vi "SGUI Assign Single String With Tags.vi"(6 "error in":errorcluster, 8 "string ref":refnum<vi>, 9 "string (empty)":string, 10 "keep last font face setup (False)":bool) -> (7 "error out":errorcluster, 11 "string ref out (copy)":refnum<vi>)   [LabVIEW 2013, in "varilib.lvlib"]
doc: "This VI parses string for tags, assigns the text to the references string object and then sets formats of the text according the tags. It supports multiline strings, i.e. various formats may be selected for each line or even part of the line. Nested tags are supported. If end tag is not found the start tag applies up to end of the whole string.\n\nSupported paired tags:\n <b></b> - bold\n <i></i> - coursive\n <u></u> - underline\n <s></s> - strikeout\n <tc=color></tc> - text color, 'color' is {black;white;red;green;gold;gray;cyan;blue} or hexa number: RRGGBB\n <sz=size></sz> - text size, 'size' is integer\n\nUnpaired tags (global for whole string):\n <bc=color> - background color, no end tag, changes color for entire string object\n <al=mode> - align mode, 'mode' is {left,center,right}\n <keep> - keep last font face setup (b,u,i,s)\n\n<keep> tag or 'keep last font face setup' input will inhibit reset of the font face setup, i.e. if the last used font face was for instance bold, next writting to the stringobject will be in the bold even without any tag specifier.\n\nText color specifier and size are always remembered from last use because default state is unknown. So when multiple sizes or colors were used previously in the string object it is necessary to write start tag with default color/size to start of the line to ensure defined states!\n\nIt ignores input error (executes anyway) however it will generate error if reference writting fails (invalid reference)."
uses:
  varilib.lvlib
  SGUI Assign String With Tags Tag.ctl
  SGUI Assign String With Tags Tag Type.ctl
  <vilib>/Utility/miscctls.llb/LVSelectionTypeDef.ctl
  <vilib>/Utility/error.llb/Error Cluster From Error Code.vi
  <vilib>/regexp/Match Regular Expression.xnode
  <vilib>/ErrorRing/Error Ring.xnode
panel:
  out "Array":bool[][](array[boolean])
  out "tag list":T1[](array[typedef])
  # "Text Tag\n\n<B> Bold </B>\n<I> Italic </I>\n<U> Underline </U>\n<S> Strikeout </S> \n<tc=color></tc> - text color, 'color' is {black;white;red;green;gold;gray;cyan;blue} or hexa number: RRGGBB\n <sz=size></sz> - text size, 'size' is integer\n\nUnpaired tags (global for whole string):\n <bc=color> - background color, no end tag, changes color for entire string object\n <al=mode> - align mode, 'mode' is {left,center,right}\n <keep> - keep last font face setup (b,u,i,s)"
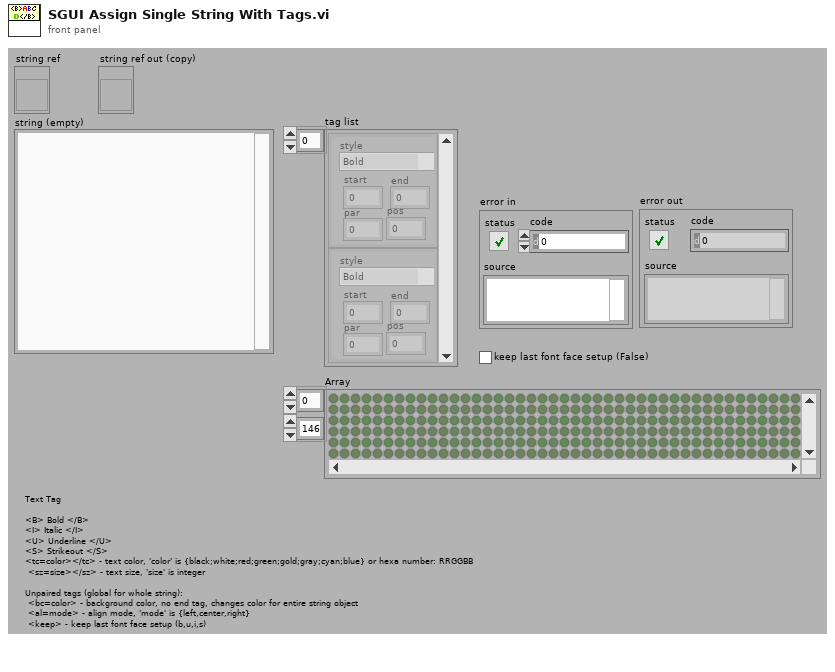
[diagram p1: front panel]
types:
  T1 = typedef "varilib.lvlib/SGUI Assign String With Tags Tag.ctl" = cluster{"pos":i32, "style":T2, "start":i32, "end":i32, "par":i32}
  T2 = typedef "varilib.lvlib/SGUI Assign String With Tags Tag Type.ctl" = enum16{"Bold", "Italic", "Underline", "Strikeout", "Text color", "Bg color", "Align", "Size", "Keep", "n/a"}
  T3 = typedef "LVSelectionTypeDef.ctl" = cluster{"Selection Start":u32, "Selection End":u32}
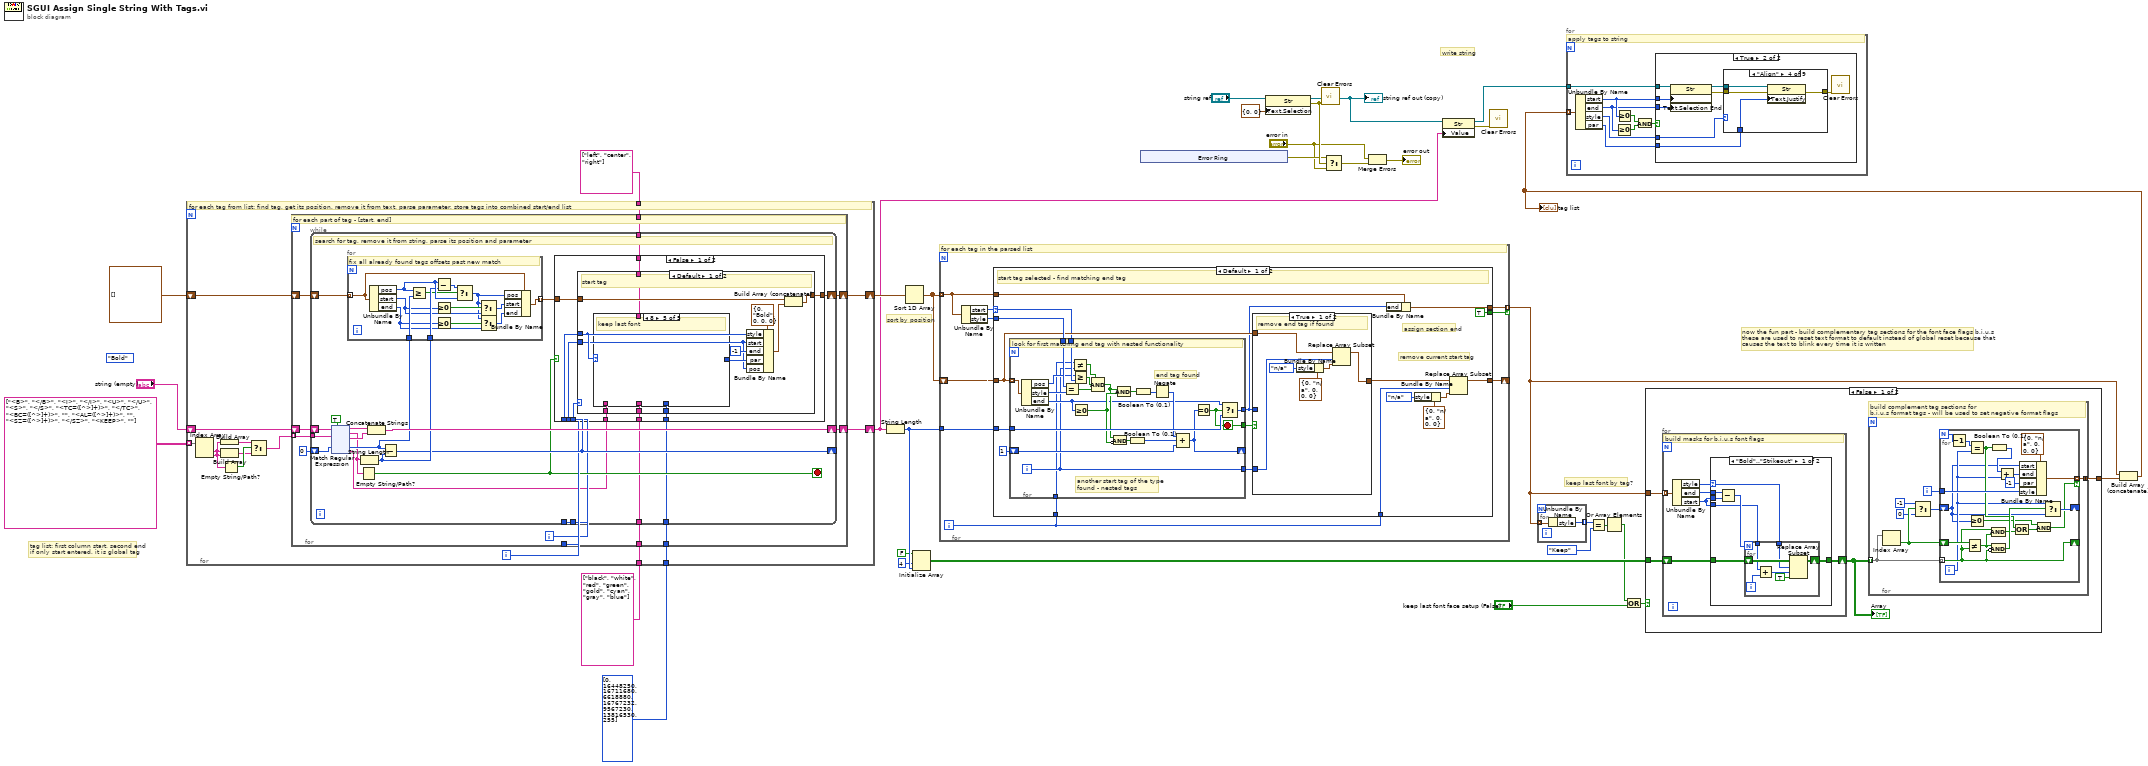
[diagram p0: block diagram]
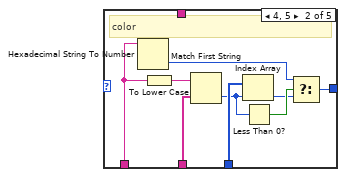
[diagram p7: hidden frame]
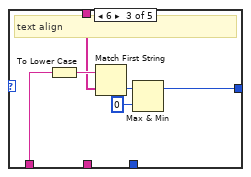
[diagram p8: hidden frame]
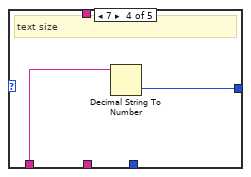
[diagram p9: hidden frame]
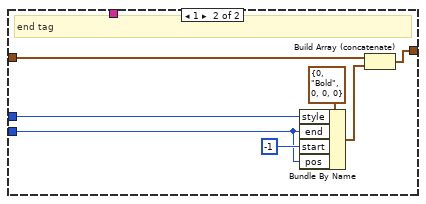
[diagram p10: hidden frame]
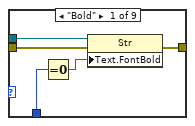
[diagram p13: hidden frame]
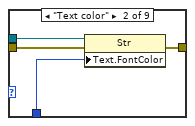
[diagram p14: hidden frame]
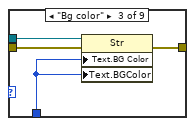
[diagram p15: hidden frame]
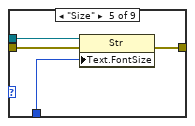
[diagram p16: hidden frame]
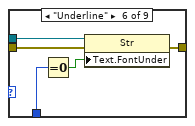
[diagram p17: hidden frame]
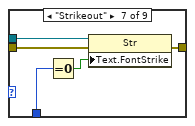
[diagram p18: hidden frame]
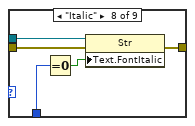
[diagram p19: hidden frame]
diagram:
  (unwired) SGUI_Assign_String_With_Tags_Tag_Type."Bold" ("style")
  # "keep last font by tag?"
  # "now the fun part - build complementary tag sections for the font face flags b,i,u,s\nthese are used to reset text format to default instead of global reset because that\ncauses the text to blink every time it is written"
  # "tag list: first column start, second end\nif only start entered, it is global tag"
  # "write string"
  # "sort by position"
  n1 = for {
    tunnel: string[][] [["<B>", "</B>"], ["<I>", "</I>"], ["<U>", "</U>"], ["<S>", "</S>"], ["<TC=([^>]+)>", "</TC>"], ["<BC=([^>]+)>", ""], ["<AL=([^>]+)>", ""], ["<SZ=([^>]+)>", "</SZ>"], ["<KEEP>", ""]] -> [w46] mode=indexing
    shift-right: [w45] -> w20
    shift-left: "string (empty)" -> [w47]
    shift-right: [w43] -> w25
    shift-left: T1[] [] -> [w44]
    tunnel: string[] ["black", "white", "red", "green", "gold", "cyan", "gray", "blue"] ("string array") -> [w41]
    tunnel: u32[] [0, 16448250, 16711680, 6618880, 16767232, 9567230, 13816530, 255] -> [w40]
    tunnel: string[] ["left", "center", "right"] ("string array") -> [w33]
    i -> [w42]
    # "for each tag from list: find tag, get its position, remove it from text, parse parameter, store tags into combined start/end list"
    n2 = Index Array(array=w46) -> (element #1=w35:string, element #2=w37:string)  [unwired: 2 in]
    n3 = Build Array(w35) -> (w34:string[])
    n4 = Build Array(w35, w37) -> (w36:string[])
    n5 = Empty String/Path?(string/path=w37) -> (empty?=w38:bool)
    n6 = Select(t=w34, s=w38, f=w36) -> (s? t:f=w39:string[])
    n7 = for {
      tunnel: w39 -> [w57] mode=indexing
      tunnel: w42 -> [w53]
      shift-right: [w52] -> w43
      shift-left: w44 -> [w54]
      shift-right: [w56] -> w45
      shift-left: w47 -> [w58]
      tunnel: w41 -> [w50]
      tunnel: w40 -> [w49]
      tunnel: w33 -> [w48]
      i -> [w51]
      # "for each part of tag - [start, end]"
      n8 = while {
        tunnel: w57 -> [w64]
        shift-right: [w70] -> _
        shift-left: 0 -> [w76]
        shift-right: [w77] -> w56
        shift-left: w58 -> [w75]
        shift-right: [w67] -> w52
        shift-left: w54 -> [w73]
        tunnel: w53 -> [w69]
        tunnel: w51 -> [w65]
        tunnel: w50 -> [w61]
        tunnel: w49 -> [w60]
        tunnel: w48 -> [w59]
        stop <- w66 stop-if-true
        # "search for tag, remove it from string, parse its position and parameter"
        n9 = xnode "Match Regular Expression"("input string"=w75, "regular expression"=w64, "offset (0)"=w76, "ignore case? (F)"=TRUE) -> ("before match"=w79:string, "whole match"=w62:string, "after match"=w78:string, "offset past match"=w72:i32, "submatch 1"=w63:string)  [unwired: 2 in, 1 out]
        n10 = Empty String/Path?(string/path=w62) -> (empty?=w66:bool)
        n11 = String Length(string=w62) -> (length=w71:i32)
        n12 = for {
          tunnel: w73 -> [w135] mode=indexing
          tunnel: w72 -> [w139]
          tunnel: w71 -> [w136]
          tunnel: [w134] -> w68 mode=indexing
          # "fix all already found tags offsets past new match"
          n13 = Unbundle By Name(w135) -> ("pos"=w137:i32, "start"=w130:i32, "end"=w127:i32)
          n14 = Greater Or Equal?(x=w137, y=w139) -> (x >= y?=w133:bool)
          n15 = Subtract(x=w137, y=w136) -> (x-y=w138:i32)
          n16 = Greater Or Equal To 0?(x=w130) -> (x >= 0?=w132:bool)
          n17 = Greater Or Equal To 0?(x=w127) -> (x >= 0?=w129:bool)
          n18 = Select(t=w138, s=w133, f=w137) -> (s? t:f=w126:i32)
          n19 = Select(t=w126, s=w132, f=w130) -> (s? t:f=w131:i32)
          n20 = Select(t=w126, s=w129, f=w127) -> (s? t:f=w128:i32)
          n21 = Bundle By Name(cluster=w135, "pos"=w126, "start"=w131, "end"=w128) -> (w134:T1)
        }
        n22 = Concatenate Strings(w79, w78) -> (w77:string)
        n23 = Subtract(x=w72, y=w71) -> (x-y=w70:i32)
        n24 = case shown="False" w66 {
          tunnel: w70 -> [w88 _]
          tunnel: w69 -> [w87 _]
          tunnel: w68 -> [w86 w125]
          tunnel: [w85 w125] -> w67
          tunnel: w65 -> [w84 _]
          tunnel: w63 -> [w83 _]
          tunnel: w61 -> [w82 _]
          tunnel: w60 -> [w81 _]
          tunnel: w59 -> [w80 _]
          frame False {
            n25 = case shown="Default" w84 {
              tunnel: w88 -> [w92 w118]
              tunnel: w87 -> [w95 w122]
              tunnel: w86 -> [w98 w121]
              tunnel: [w96 w119] -> w85
              tunnel: w83 -> [w94 _]
              tunnel: w82 -> [w91 _]
              tunnel: w81 -> [w90 _]
              tunnel: w80 -> [w89 _]
              frame Default {
                # "start tag"
                n26 = case shown="8" w95 {
                  tunnel: w94 -> [_ w108 w115 w117 _]
                  tunnel: [_ w106 w110 w116 _] -> w93
                  tunnel: w91 -> [_ w109 _ _ _]
                  tunnel: w90 -> [_ w107 _ _ _]
                  tunnel: w89 -> [_ _ w113 _ _]
                  frame Default {
                  }
                  frame 4, 5 {
                    # "color"
                    n27 = Hexadecimal String To Number(string=w108) -> (number=w103:u32)  [unwired: 2 in, 1 out]
                    n28 = To Lower Case(string=w108) -> (all lower case string=w101:string)
                    n29 = Match First String(2:w109, 3:w101) -> (0:w105:i32)  [unwired: 1 out]
                    n30 = Index Array(array=w107, index=w105) -> (element=w102:u32)
                    n31 = Less Than 0?(x=w105) -> (x < 0?=w104:bool)
                    n32 = Select(t=w103, s=w104, f=w102) -> (s? t:f=w106:u32)
                  }
                  frame 6 {
                    # "text align"
                    n33 = To Lower Case(string=w115) -> (all lower case string=w114:string)
                    n34 = Match First String(2:w113, 3:w114) -> (0:w112:i32)  [unwired: 1 out]
                    n35 = Max & Min(x=w112, y=0) -> (max(x,y)=w110:i32)  [unwired: 1 out]
                  }
                  frame 7 {
                    # "text size"
                    n36 = Decimal String To Number(string=w117) -> (number=w116:i32)  [unwired: 2 in, 1 out]
                  }
                  frame 8 {
                    # "keep last font"
                  }
                }
                n37 = Bundle By Name(cluster=T1 {"pos"=0, "style"=enum."Bold", "start"=0, "end"=0, "par"=0} ("tag"), "style"=w95, "start"=w92, "end"=-1, "par"=w93, "pos"=w92) -> (w97:T1)
                n38 = Build Array (concatenate)(w98, w97) -> (w96:T1[])
              }
              frame 1 {
                # "end tag"
                n39 = Bundle By Name(cluster=T1 {"pos"=0, "style"=enum."Bold", "start"=0, "end"=0, "par"=0} ("tag"), "style"=w122, "end"=w118, "start"=-1 ("end"), "pos"=w118) -> (w120:T1)
                n40 = Build Array (concatenate)(w121, w120) -> (w119:T1[])
              }
            }
          }
          frame True {
          }
        }
      }
    }
  }
  n41 = String Length(string=w20) -> (length=w18:i32)
  n42 = Sort 1D Array(array=w25) -> (sorted array=w29:T1[])
  n43 = Initialize Array(FALSE, 4 ("dimension size"), w18) -> (w15:bool[][])
  n44 = for {
    tunnel: w29 -> [w260] mode=indexing
    shift-right: [w261] -> _
    shift-left: w29 -> [w263]
    tunnel: [w259] -> w12 mode=indexing if=w258
    tunnel: w18 -> [w257]
    i -> [w256]
    # "for each tag in the parsed list"
    n45 = Unbundle By Name(w260) -> ("start"=w264:i32, "style"=w262:T2)
    n46 = case shown="Default" w264 {
      selector: w264 -> [w266 _]
      tunnel: w263 -> [w281 w313]
      tunnel: w262 -> [w282 _]
      tunnel: [w271 w313] -> w261
      tunnel: w260 -> [w269 w314]
      tunnel: [w268 w314] -> w259
      tunnel: [TRUE _] -> w258
      tunnel: w257 -> [w278 _]
      tunnel: w256 -> [w270 _]
      tunnel: w256 -> [w265 _]
      frame Default {
        # "assign section end"
        # "remove current start tag"
        # "start tag selected - find matching end tag"
        n47 = for {
          tunnel: w281 -> [w312] mode=indexing
          tunnel: w282 -> [w310]
          tunnel: [w309] -> w267
          tunnel: [w292] -> w280
          tunnel: w278 -> [w308]
          shift-right: [w301] -> _
          shift-left: i16 1 -> [w303]
          tunnel: [w299] -> w276
          tunnel: w266 -> [w298]
          tunnel: w265 -> [w291]
          i -> [w292]
          stop <- w299 stop-if-true
          # "another start tag of the type\nfound - nested tags"
          # "end tag found"
          # "look for first matching end tag with nested functionality"
          n48 = Unbundle By Name(w312) -> ("pos"=w293:i32, "style"=w311:T2, "end"=w294:i32)
          n49 = Equal?(x=w310, y=w311) -> (x = y?=w296:bool)
          n50 = Not Equal?(x=w291, y=w292) -> (x != y?=w290:bool)
          n51 = Greater Or Equal?(x=w293, y=w298) -> (x >= y?=w297:bool)
          n52 = Greater Or Equal To 0?(x=w294) -> (x >= 0?=w307:bool)
          n53 = Compound Arithmetic op=AND(w290, w297, w296) -> (w295:bool)
          n54 = Compound Arithmetic op=AND(w295, invert w307) -> (w306:bool)
          n55 = Compound Arithmetic op=AND(w295, w307) -> (w305:bool)
          n56 = Boolean To (0,1)(Boolean=w306) -> (0, 1=w304:i16)
          n57 = Boolean To (0,1)(Boolean=w305) -> (0, 1=w302:i16)
          n58 = Negate(x=w302) -> (-x=w300:i16)
          n59 = Compound Arithmetic op=ADD(w300, w304, w303) -> (w301:i16)
          n60 = Equal To 0?(x=w301) -> (x = 0?=w299:bool)
          n61 = Select(t=w294, s=w299, f=w308) -> (s? t:f=w309:i32)
        }
        n62 = case shown="True" w276 {
          tunnel: w281 -> [w288 w289]
          tunnel: w280 -> [w287 _]
          tunnel: [w286 w289] -> w272
          tunnel: w267 -> [_ _]
          frame True {
            # "remove end tag if found"
            n63 = Bundle By Name(cluster=T1 {"pos"=0, "style"=enum."n/a", "start"=0, "end"=0, "par"=0} ("new element/subarray"), "style"=SGUI_Assign_String_With_Tags_Tag_Type."n/a") -> (w285:T1)
            n64 = Replace Array Subset(array=w288, new element=w285, index=w287) -> (w286:T1[])
          }
          frame False {
          }
        }
        n65 = Bundle By Name(cluster=w269, "end"=w267) -> (w268:T1)
        n66 = Bundle By Name(cluster=T1 {"pos"=0, "style"=enum."n/a", "start"=0, "end"=0, "par"=0} ("new element/subarray"), "style"=SGUI_Assign_String_With_Tags_Tag_Type."n/a") -> (w273:T1)
        n67 = Replace Array Subset(array=w272, new element=w273, index=w270) -> (w271:T1[])
      }
      frame -1 {
      }
    }
  }
  n68 = xnode "Error Ring"() -> ("error out"=w2:errorcluster)
  n69 = property class="Str"(reference="string ref", "Text.Selection"=T3 {"Selection Start"=0, "Selection End"=0}) -> (reference out=w19:refnum<vi>, error out=w3:errorcluster)  [unwired: 1 in]
  "string ref out (copy)" <- w19
  n70 = call <vilib>:"Clear Errors.vi"("error in (no error)"=w3) -> ()  [unwired: 6 in, 1 out]
  n71 = Select(t=w2, s=w3, f="error in") -> (s? t:f=w4:errorcluster)
  n72 = Merge Errors("error in", w4) -> (→"error out":errorcluster)
  n73 = property class="Str"(reference=w19, "Value"=w20) -> (reference out=w21:refnum<vi>, error out=w22:errorcluster)  [unwired: 1 in]
  n74 = call <vilib>:"Clear Errors.vi"("error in (no error)"=w22) -> ()  [unwired: 6 in, 1 out]
  n75 = for {
    tunnel: w12 -> [w316] mode=indexing
    tunnel: [w315] -> w11 mode=indexing
    n76 = Unbundle By Name(w316) -> ("style"=w315:T2)
  }
  n77 = Equal?(x=w11, y=SGUI_Assign_String_With_Tags_Tag_Type."Keep" ("style")) -> (x = y?=w9:bool[])
  n78 = Or Array Elements(Boolean array=w9) -> (logical OR=w8:bool)
  n79 = Compound Arithmetic op=OR(w8, "keep last font face setup (False)") -> (w6:bool)
  n80 = case shown="False" w6 {
    tunnel: w15 -> [w320 _]
    tunnel: [w318 _] -> w14
    tunnel: w12 -> [w317 _]
    frame False {
      n81 = for {
        tunnel: w317 -> [w353] mode=indexing
        shift-right: [w348] -> w319
        shift-left: w320 -> [w351]
        # "build masks for b,i,u,s font flags"
        n82 = Unbundle By Name(w353) -> ("style"=w352:T2, "end"=w350:i32, "start"=w349:i32)
        n83 = case shown="\"Bold\"..\"Strikeout\"" w352 {
          selector: w352 -> [w357 _]
          tunnel: w351 -> [w360 w368]
          tunnel: w350 -> [w359 _]
          tunnel: w349 -> [w358 _]
          tunnel: w349 -> [w355 _]
          tunnel: [w354 w368] -> w348
          frame "Bold".."Strikeout" {
            n84 = Subtract(x=w359, y=w358) -> (x-y=w356:i32)
            n85 = for {
              N: w356 -> [_]
              tunnel: w357 -> [w365]
              shift-right: [w363] -> w354
              shift-left: w360 -> [w367]
              tunnel: w355 -> [w361]
              i -> [w366]
              n86 = Add(x=w361, y=w366) -> (x+y=w362:i32)
              n87 = Replace Array Subset(array=w367, new element=TRUE ("new element/subarray"), index (row)=w365, index (col)=w362) -> (w363:bool[][])
            }
          }
          frame Default {
          }
        }
      }
      "Array" <- w319
      n88 = for {
        tunnel: w319 -> [w327] mode=indexing
        tunnel: [w325] -> w318 mode=concatenating
        i -> [w326]
        # "build complement tag sections for\nb,i,u,s format tags - will be used to set negative format flags"
        n89 = Index Array(array=w327) -> (element=w323:bool)  [unwired: 1 in]
        n90 = Select(t=-1, s=w323, f=0) -> (s? t:f=w324:i32)
        n91 = for {
          N -> [w339]
          tunnel: w327 -> [w340] mode=indexing
          shift-right: [w340] -> _
          shift-left: w323 -> [w347]
          shift-right: [w345] -> _
          shift-left: w324 -> [w331]
          tunnel: w326 -> [w342]
          tunnel: [w341] -> w325 mode=indexing if=w328
          i -> [w332]
          n92 = Decrement(x=w339) -> (x-1=w338:i32)
          n93 = Not Equal?(x=w347, y=w340) -> (x != y?=w337:bool)
          n94 = Greater Or Equal To 0?(x=w331) -> (x >= 0?=w329:bool)
          n95 = Equal?(x=w338, y=w332) -> (x = y?=w335:bool)
          n96 = Boolean To (0,1)(Boolean=w335) -> (0, 1=w333:i16)
          n97 = Compound Arithmetic op=AND(w340, w337) -> (w336:bool)
          n98 = Compound Arithmetic op=AND(w337, invert w340) -> (w346:bool)
          n99 = Add(x=w333, y=w332) -> (x+y=w334:i32)
          n100 = Compound Arithmetic op=OR(w335, w336) -> (w330:bool)
          n101 = Bundle By Name(cluster=T1 {"pos"=0, "style"=enum."n/a", "start"=0, "end"=0, "par"=0} ("new element/subarray"), "start"=w331, "end"=w334, "par"=-1, "style"=w342) -> (w341:T1)
          n102 = Compound Arithmetic op=AND(w329, w330) -> (w328:bool)
          n103 = Select(t=w332, s=w346, f=w331) -> (s? t:f=w345:i32)
        }
      }
    }
    frame True {
    }
  }
  n104 = Build Array (concatenate)(w12, w14) -> (w13:T1[])
  "tag list" <- w13
  n105 = for {
    tunnel: w13 -> [w377] mode=indexing
    tunnel: w21 -> [w371]
    # "apply tags to string"
    n106 = Unbundle By Name(w377) -> ("start"=w373:i32, "end"=w372:i32, "style"=w370:T2, "par"=w369:i32)
    n107 = Greater Or Equal To 0?(x=w372) -> (x >= 0?=w375:bool)
    n108 = Greater Or Equal To 0?(x=w373) -> (x >= 0?=w376:bool)
    n109 = And(x=w376, y=w375) -> (x .and. y?=w374:bool)
    n110 = case shown="True" w374 {
      tunnel: w371 -> [_ w385]
      tunnel: w373 -> [_ w384]
      tunnel: w372 -> [_ w383]
      tunnel: w370 -> [_ w381]
      tunnel: w369 -> [_ w380]
      frame False {
      }
      frame True {
        n111 = property class="Str"(reference=w385, "Text.Selection Start"=w384, "Text.Selection End"=w383) -> (reference out=w382:refnum<vi>, error out=w379:errorcluster)  [unwired: 1 in]
        n112 = case shown="\"Align\"" w381 {
          tunnel: w382 -> [w390 w394 w398 w402 w406 w411 w416 w421 _]
          tunnel: w380 -> [w387 w393 w397 w401 w405 w407 w412 w417 _]
          tunnel: w379 -> [w389 w392 w396 w400 w404 w410 w415 w420 w422]
          tunnel: [w388 w391 w395 w399 w403 w409 w414 w419 w422] -> w378
          frame "Bold" {
            n113 = Equal To 0?(x=w387) -> (x = 0?=w386:bool)
            n114 = property class="Str"(reference=w390, error in=w389, "Text.FontBold"=w386) -> (error out=w388:errorcluster)  [unwired: 1 out]
          }
          frame "Text color" {
            n115 = property class="Str"(reference=w394, error in=w392, "Text.FontColor"=w393) -> (error out=w391:errorcluster)  [unwired: 1 out]
          }
          frame "Bg color" {
            n116 = property class="Str"(reference=w398, error in=w396, "Text.BG Color"=w397, "Text.BGColor"=w397) -> (error out=w395:errorcluster)  [unwired: 1 out]
          }
          frame "Align" {
            n117 = property class="Str"(reference=w402, error in=w400, "Text.Justify"=w401) -> (error out=w399:errorcluster)  [unwired: 1 out]
          }
          frame "Size" {
            n118 = property class="Str"(reference=w406, error in=w404, "Text.FontSize"=w405) -> (error out=w403:errorcluster)  [unwired: 1 out]
          }
          frame "Underline" {
            n119 = Equal To 0?(x=w407) -> (x = 0?=w408:bool)
            n120 = property class="Str"(reference=w411, error in=w410, "Text.FontUnder"=w408) -> (error out=w409:errorcluster)  [unwired: 1 out]
          }
          frame "Strikeout" {
            n121 = Equal To 0?(x=w412) -> (x = 0?=w413:bool)
            n122 = property class="Str"(reference=w416, error in=w415, "Text.FontStrike"=w413) -> (error out=w414:errorcluster)  [unwired: 1 out]
          }
          frame "Italic" {
            n123 = Equal To 0?(x=w417) -> (x = 0?=w418:bool)
            n124 = property class="Str"(reference=w421, error in=w420, "Text.FontItalic"=w418) -> (error out=w419:errorcluster)  [unwired: 1 out]
          }
          frame Default {
          }
        }
        n125 = call <vilib>:"Clear Errors.vi"("error in (no error)"=w378) -> ()  [unwired: 6 in, 1 out]
      }
    }
  }
